vi "OpenScan FPGA Host.vi"() -> ()   [LabVIEW 2015]
uses:
  <vilib>/rvi/Emulation/niFpgaGetClockAttributes.vi
  <vilib>/rvi/Emulation/niFpgaSctlEmulationGetInTimedLoop.vi
  <vilib>/rvi/Emulation/niFpgaEmulationReportErrorSimple.vi
  <vilib>/rvi/Emulation/niFpgaProcessEmulError.vi
  <vilib>/rvi/Emulation/niFpgaCriticalErrorInLSC.vi
panel:
  in  "Ready to Scan":bool
  out "Frame acquisition finish?":bool
  out "loop count":i32
  out "Display_frames done":i32
  out "Averaged data address":u32
  out "Frame imaging data averaged?":bool
  out "Averaged image displayed?":bool
  out "Image averaging done?":bool
  in  "Kalman gain":fxp<+,16,1>=0.1015625
  in  "Filter gain":fxp<+,16,0>=0.8000030517578125
  in  "Frame number":i32
  out "Line clock":bool
  out "Pixel clock (Indicator)":bool
  out "Data":u32
  out "Galvo signal readed":u32
  out "Request address":u32
  out "Frame waveform output finish?":bool
  in  "Pixel clock_pulse width(tick)":i32
  in  "Resolution":i32
  in  "Elements per line":i32
  in  "Num of elements":u32
  in  "Pixel time (tick)":i32
  in  "Num of undershoot":i32
  in  "Pixel pulse_initial delay":i32
  in  "Frame retrace time":u32 caption="Frame retrace time (ms)"
  in  "Samples per frame control":u32=262144
  in  "Number of frames":i32
  in  "Max DRAM address":u32
  out "Frame Galvo signal write done?":bool
  out "Write DRAM done?":bool
  in  "Total elements":u32=512000
  in  "Write DRAM enable?":bool
  in  "max addr":u32=1000
  in  "Write Frame Galvo signal?":bool
  in  "Current":T1(ring)
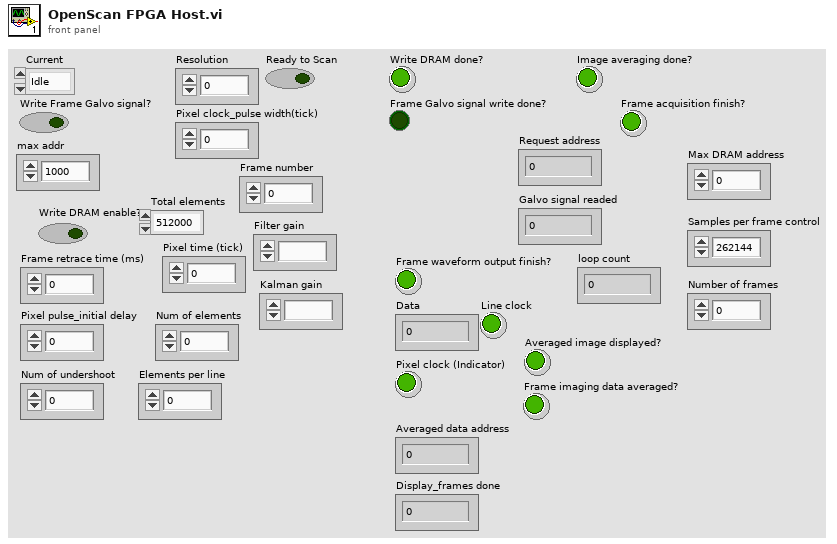
[diagram p1: front panel]
types:
  T1 = enum16{"Idle", "Init", "Write", "Scan", "Blank", "Stop"}
  T2 = cluster{"Max DRAM address":u32, "Samples per frame control":u32, "Number of frames":i32}
  T3 = cluster{"Write Frame Galvo signal?":bool, "max addr":u32, "Write DRAM enable?":bool, "Total elements":u32}
  T4 = cluster{"Frame retrace time":u32, "Pixel pulse_initial delay":i32, "Num of undershoot":i32, "Pixel time (tick)":i32, "Num of elements":u32, "Elements per line":i32, "Resolution":i32, "Pixel clock_pulse width(tick)":i32}
  T5 = cluster{"Frame number":i32, "Filter gain":fxp<+,16,0>, "Kalman gain":fxp<+,16,1>}
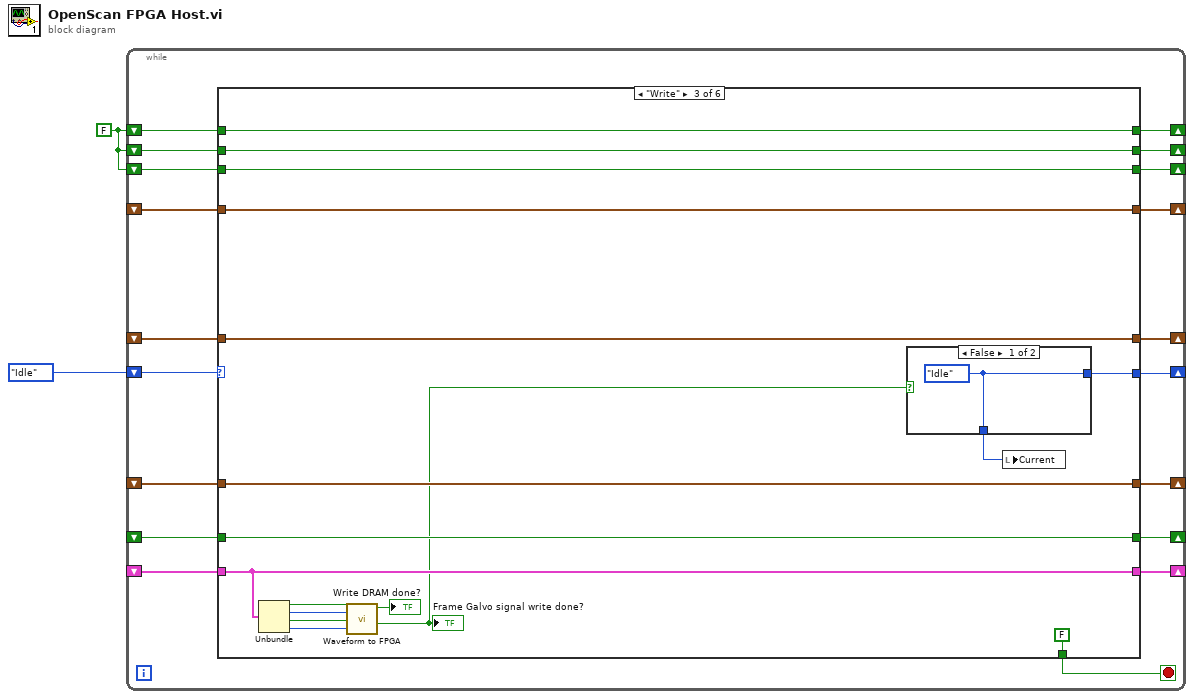
[diagram p0: block diagram]
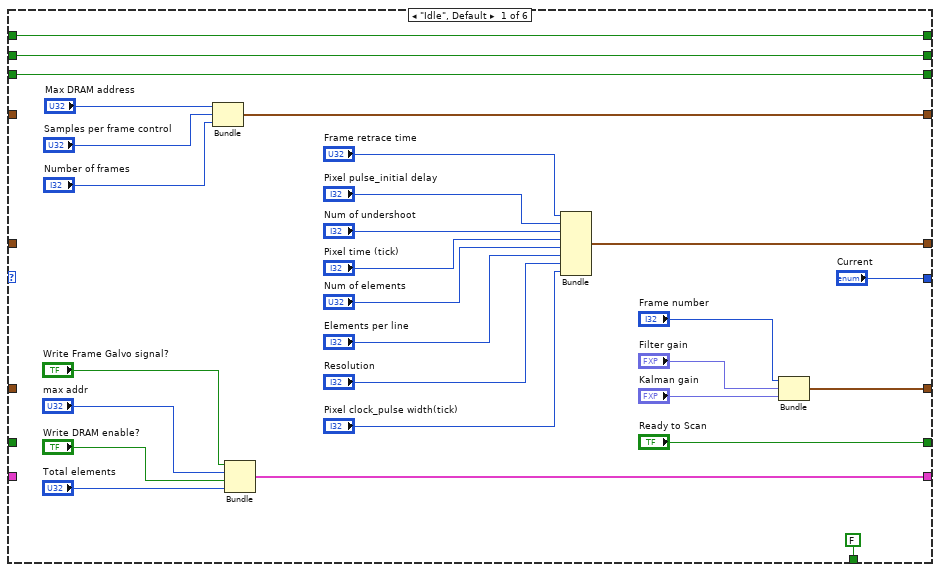
[diagram p2: hidden frame]
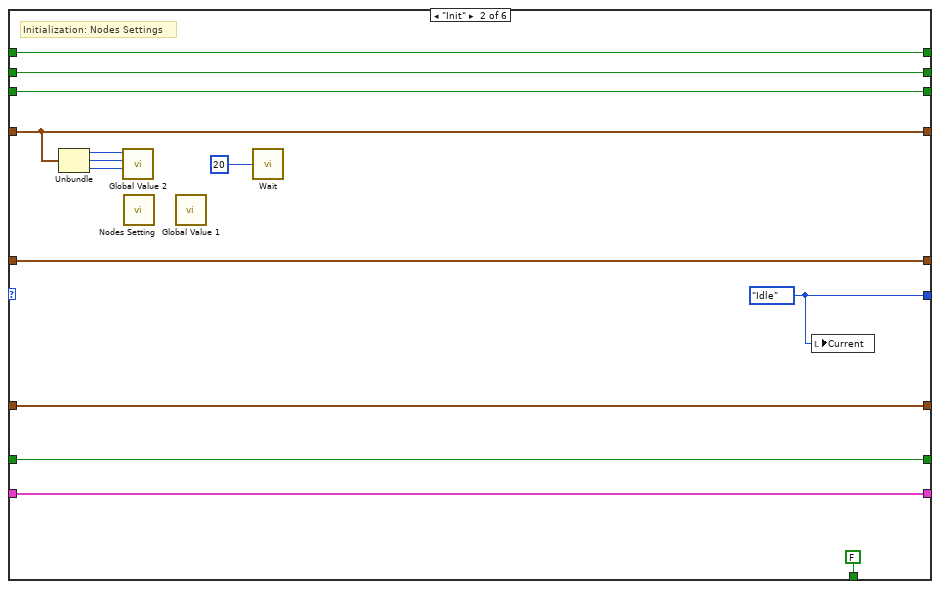
[diagram p3: hidden frame]
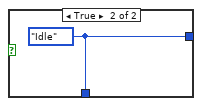
[diagram p4: hidden frame]
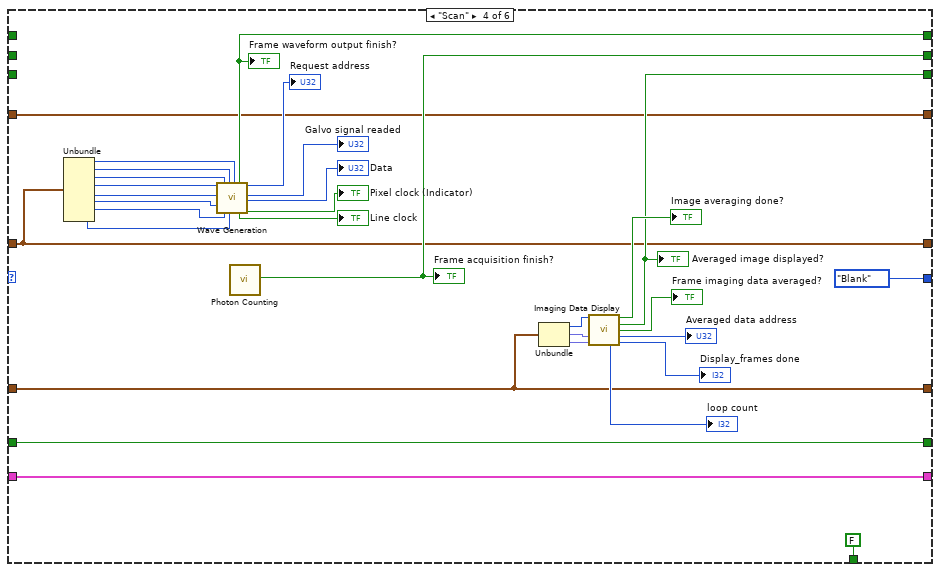
[diagram p5: hidden frame]
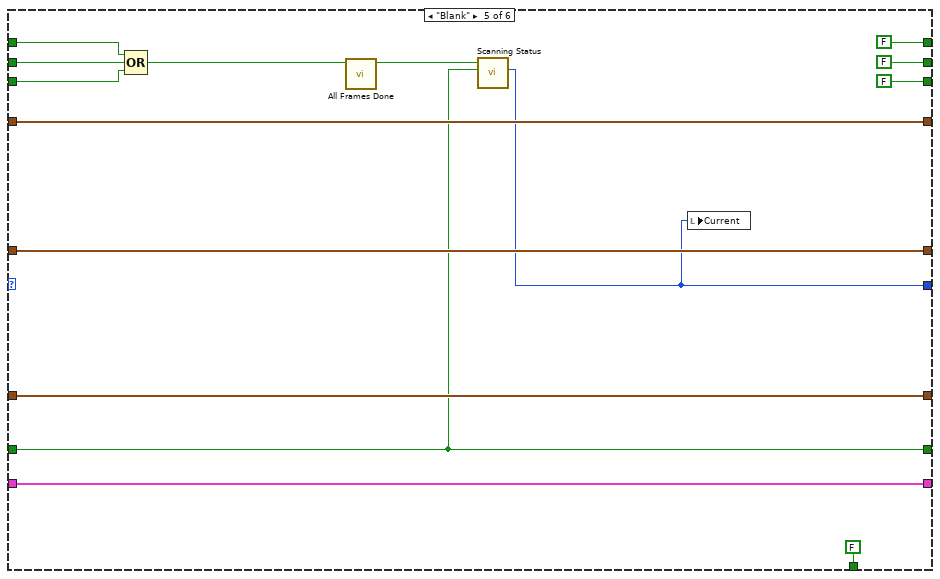
[diagram p6: hidden frame]
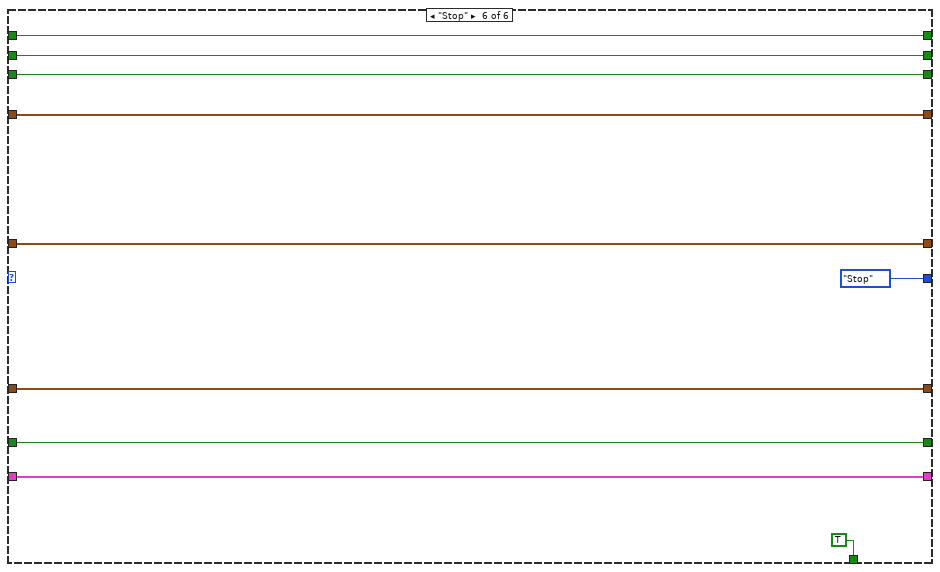
[diagram p7: hidden frame]
diagram:
  w1 = FALSE ("Frame waveform output finish?")
  n1 = while {
    shift-right: [w20] -> _
    shift-left: T1."Idle" -> [w21]
    shift-right: [w19] -> _
    shift-left: w1 -> [w16]
    shift-right: [w18] -> _
    shift-left: w1 -> [w15]
    shift-right: [w17] -> _
    shift-left: w1 -> [w14]
    shift-right: [w12] -> _
    shift-left: _ -> [w11]
    shift-right: [w10] -> _
    shift-left: _ -> [w6]
    shift-right: [w9] -> _
    shift-left: _ -> [w8]
    shift-right: [w7] -> _
    shift-left: _ -> [w5]
    shift-right: [w4] -> _
    shift-left: _ -> [w3]
    stop <- w13 stop-if-true
    n2 = case shown="\"Write\"" w21 {
      tunnel: ["Current" w50 w79 T1."Blank" ("Current") w114 T1."Stop" ("Next Status")] -> w20
      tunnel: [w48 w62 w78 w102 FALSE ("Frame waveform output finish?") w138] -> w19
      tunnel: [w47 w61 w77 w101 FALSE ("Frame acquisition finish?") w137] -> w18
      tunnel: [w46 w60 w76 w100 FALSE ("Averaged image displayed?") w136] -> w17
      tunnel: w16 -> [w48 w62 w78 _ w128 w138]
      tunnel: w15 -> [w47 w61 w77 _ w127 w137]
      tunnel: w14 -> [w46 w60 w76 _ w126 w136]
      tunnel: [FALSE FALSE FALSE FALSE FALSE TRUE] -> w13
      tunnel: [w41 w55 w69 w83 w119 w133] -> w12
      tunnel: w11 -> [_ w55 w69 w83 w119 w133]
      tunnel: [w28 w54 w68 w84 w118 w132] -> w10
      tunnel: [w27 w51 w70 w85 w115 w129] -> w9
      tunnel: w8 -> [_ w51 w70 w85 w115 w129]
      tunnel: [w23 w53 w67 w90 w117 w131] -> w7
      tunnel: w6 -> [_ w54 w68 w84 w118 w132]
      tunnel: w5 -> [_ w53 w67 w90 w117 w131]
      tunnel: ["Ready to Scan" w52 w66 w86 w116 w130] -> w4
      tunnel: w3 -> [_ w52 w66 w86 w116 w130]
      frame "Idle", Default {
        n3 = Bundle("Max DRAM address"="Max DRAM address", "Samples per frame control"="Samples per frame control", "Number of frames"="Number of frames") -> (w41:T2)  [unwired: 1 in]
        n4 = Bundle("Write Frame Galvo signal?"="Write Frame Galvo signal?", "max addr"="max addr", "Write DRAM enable?"="Write DRAM enable?", "Total elements"="Total elements") -> (w27:T3)  [unwired: 1 in]
        n5 = Bundle("Frame retrace time"="Frame retrace time", "Pixel pulse_initial delay"="Pixel pulse_initial delay", "Num of undershoot"="Num of undershoot", "Pixel time (tick)"="Pixel time (tick)", "Num of elements"="Num of elements", "Elements per line"="Elements per line", "Resolution"="Resolution", "Pixel clock_pulse width(tick)"="Pixel clock_pulse width(tick)") -> (w28:T4)  [unwired: 1 in]
        n6 = Bundle("Frame number"="Frame number", "Filter gain"="Filter gain", "Kalman gain"="Kalman gain") -> (w23:T5)  [unwired: 1 in]
      }
      frame "Init" {
        w50 = T1."Idle" ("Next Status")
        # "Initialization: Nodes Settings"
        n7 = Unbundle(w55) -> ("Max DRAM address"=w58:u32, "Samples per frame control"=w57:u32, "Number of frames"=w56:i32)
        n8 = call "Global Value 2.vi"("Number of frames"=w56, "Samples per frame control"=w57, "Max DRAM address"=w58) -> ()  [unwired: 9 in]
        n9 = call "Nodes Setting.vi"() -> ()  [unwired: 12 in]
        n10 = call "Global Value 1.vi"() -> ()  [unwired: 12 in]
        n11 = call "Wait"("Count(mSec)"=u32 20) -> ()  [unwired: 1 out]
        n12 = local write "Current"(w50) -> ()
      }
      frame "Write" {
        n13 = Unbundle(w70) -> ("Write Frame Galvo signal?"=w74:bool, "max addr"=w73:u32, "Write DRAM enable?"=w72:bool, "Total elements"=w71:u32)
        n14 = call "Waveform to FPGA.vi"("Write Frame Galvo signal?"=w74, "max addr"=w73, "Write DRAM enable?"=w72, "Total elements"=w71) -> ("Write DRAM done?"=→"Write DRAM done?":bool, "Frame Galvo signal write done?"=w65:bool)  [unwired: 5 in]
        "Frame Galvo signal write done?" <- w65
        n15 = case shown="False" w65 {
          tunnel: [w81 w82] -> w79
          tunnel: [w81 w82] -> w64
          frame False {
            w81 = T1."Idle" ("Current")
          }
          frame True {
            w82 = T1."Idle" ("Current")
          }
        }
        n16 = local write "Current"(w64) -> ()
      }
      frame "Scan" {
        n17 = Unbundle(w84) -> ("Frame retrace time"=w98:u32, "Pixel pulse_initial delay"=w97:i32, "Num of undershoot"=w96:i32, "Pixel time (tick)"=w95:i32, "Num of elements"=w94:u32, "Elements per line"=w93:i32, "Resolution"=w92:i32, "Pixel clock_pulse width(tick)"=w91:i32)
        n18 = call "Wave Generation.vi"("Pixel time (tick)"=w95, "Num of elements"=w94, "Elements per line"=w93, "Num of undershoot"=w96, "Resolution"=w92, "Pixel pulse_initial delay"=w97, "Pixel clock_pulse width(tick)"=w91, "Frame retrace time"=w98) -> ("Frame waveform output finish?"=w102:bool, "Line clock"=→"Line clock":bool, "Request address"=→"Request address":u32, "Galvo signal readed"=→"Galvo signal readed":u32, "Data"=→"Data":u32, "Pixel clock"=→"Pixel clock (Indicator)":bool)  [unwired: 6 in]
        "Frame waveform output finish?" <- w102
        n19 = call "Photon Counting.vi"() -> ("Frame acquisition finish?"=w101:bool)  [unwired: 19 in]
        "Frame acquisition finish?" <- w101
        n20 = Unbundle(w90) -> ("Frame number"=w89:i32, "Filter gain"=w88:fxp<+,16,0>, "Kalman gain"=w87:fxp<+,16,1>)
        n21 = call "Imaging Data Display.vi"("Frame number"=w89, "Filter gain"=w88, "Kalman gain"=w87) -> ("Image averaging done?"=→"Image averaging done?":bool, "Averaged image displayed?"=w100:bool, "Frame imaging data Averaged?"=→"Frame imaging data averaged?":bool, "Averaged data address"=→"Averaged data address":u32, "loop count"=→"loop count":i32, "Display_frames done"=→"Display_frames done":i32)  [unwired: 7 in]
        "Averaged image displayed?" <- w100
      }
      frame "Blank" {
        n22 = Compound Arithmetic op=OR ("复合运算")(w128, w127, w126) -> (w125:bool)
        n23 = call "All Frames Done.vi"("Done in"=w125) -> ("Done out"=w124:bool)  [unwired: 10 in]
        n24 = call "Scanning Status.vi"("Ready to Scan"=w116, "Done out"=w124) -> ("Next Status"=w114:T1)  [unwired: 9 in]
        n25 = local write "Current"(w114) -> ()
      }
      frame "Stop" {
      }
    }
  }
